vi "ex14-9.vi"() -> ()   [LabVIEW 2014]
uses:
  <vilib>/NXT/Subs/MotorOutput.ctl
  <vilib>/NXT/Dual Mode Library/Motors/MotorDistance_Single.vi
panel:
  out "X-Y二進位顯示":dbl[](array[numeric])
  out "X+Y二進位顯示":dbl[](array[numeric])
  out "X-Y":dbl
  out "X+Y":dbl
  in  "減":bool
  in  "Y":dbl
  in  "X":dbl
  out "溢位?4096":bool
  out "溢位?4096":bool
  in  "加":bool
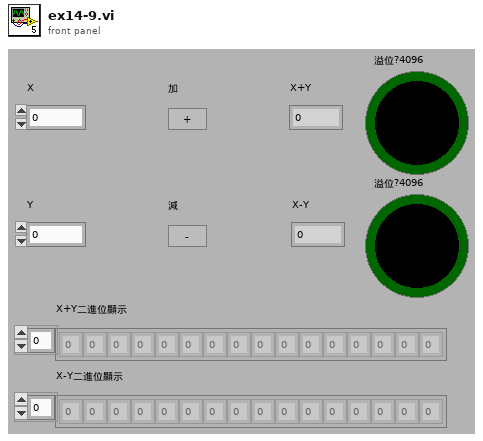
[diagram p1: front panel]
types:
  T1 = typedef "MotorOutput.ctl" = u8
  T2 = typedef "LVHSConnector.ctl" = refnum<class "BrickReference.lvclass">
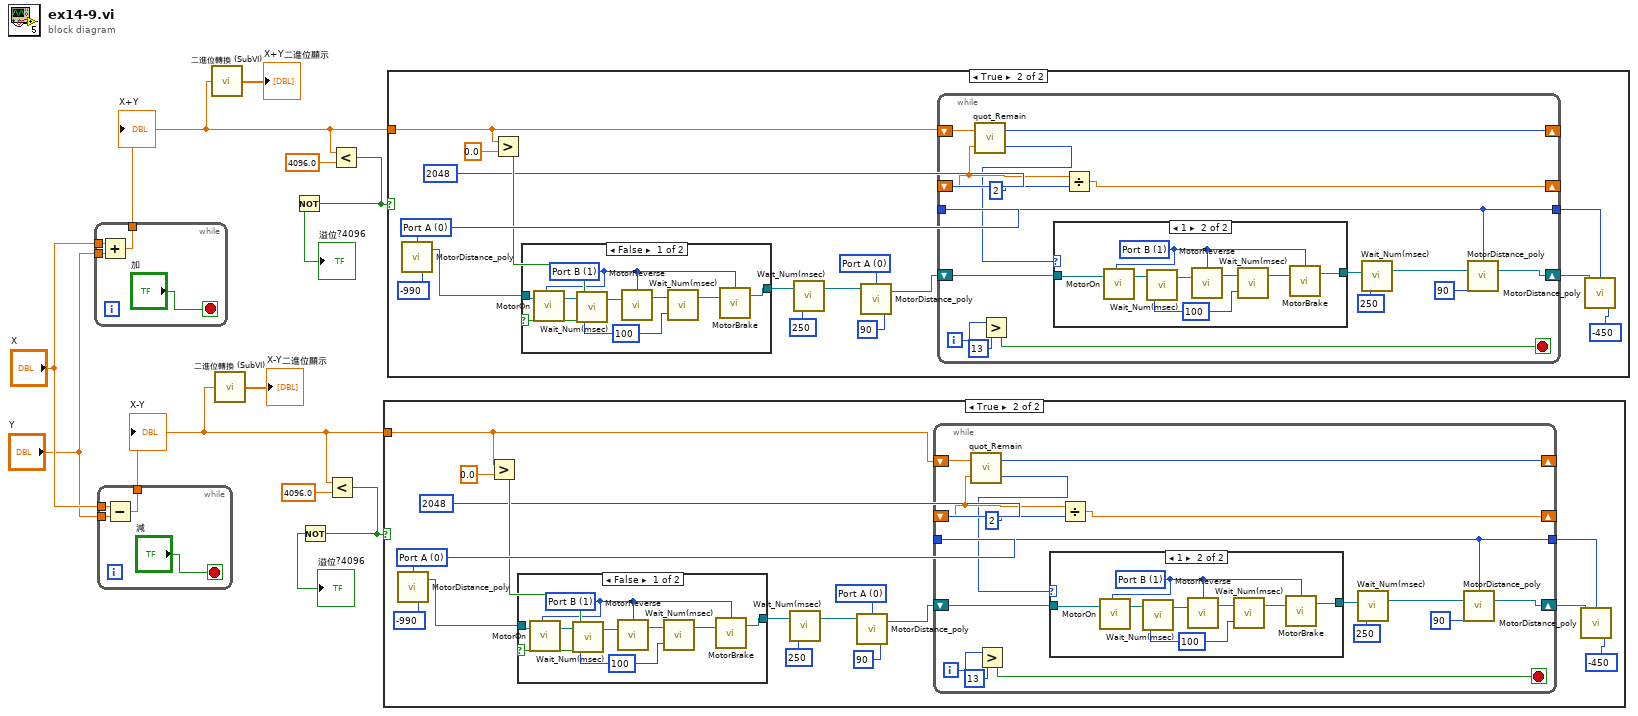
[diagram p0: block diagram]
diagram:
  n1 = while {
    tunnel: [w15] -> w4
    tunnel: "X" -> [w14]
    tunnel: "Y" -> [w13]
    stop <- "加" stop-if-true
    n2 = Add(x=w14, y=w13) -> (x+y=w15:dbl)
  }
  "X+Y" <- w4
  n3 = while {
    tunnel: [w19] -> w1
    tunnel: "X" -> [w18]
    tunnel: "Y" -> [w17]
    stop <- "減" stop-if-true
    n4 = Subtract(x=w18, y=w17) -> (x-y=w19:dbl)
  }
  "X-Y" <- w1
  n5 = call "二進位轉換 (SubVI).vi"("十進位"=w4) -> ("二進位"=→"X+Y二進位顯示":dbl[])
  n6 = call "二進位轉換 (SubVI).vi"("十進位"=w1) -> ("二進位"=→"X-Y二進位顯示":dbl[])
  n7 = Less?(x=w1, y=4096.0) -> (x < y?=w9:bool)
  n8 = Not(x=w9) -> (.not. x?=→"溢位?4096":bool)
  n9 = Less?(x=w4, y=4096.0) -> (x < y?=w11:bool)
  n10 = Not(x=w11) -> (.not. x?=→"溢位?4096":bool)
  n11 = case shown="True" w9 {
    tunnel: w1 -> [_ w21]
    frame False {
    }
    frame True {
      w23 = T1 0 items=["Port A", "Port B", "Port C", "All Ports"] ("Output Port (All Ports)")
      w33 = T1 0 items=["Port A", "Port B", "Port C", "All Ports"] ("Output Port (All Ports)")
      n12 = call-poly <vilib>:"MotorDistance_poly.vi"("Angle of Rotation (360)"=-990 ("Distance (100)"), "Output Port (All Ports)"=w33) -> ("NXT/EV3"=w29:T2)  [unwired: 2 in]
      n13 = Greater?(x=w21, y=0.0) -> (0:w30:bool)
      n14 = case shown="False" w30 {
        tunnel: w29 -> [w37 w45]
        tunnel: [w38 w45] -> w24
        frame False {
          w44 = u32 100 ("Time (100 msec)")
          w39 = T1 1 items=["Port A", "Port B", "Port C", "All Ports"] ("Output Port (All Ports)")
          n15 = call <vilib>:"MotorOn.vi"("NXT/EV3"=w37, "Output Port (All Ports)"=w39) -> ("NXT/EV3"=w43:T2)  [unwired: 2 in]
          n16 = call <vilib>:"Wait_Num(msec).vi"("Time (100 msec)"=w44, "NXT/EV3"=w43) -> ("NXT/EV3"=w42:T2)  [unwired: 2 in]
          n17 = call <vilib>:"MotorReverse.vi"("NXT/EV3"=w42, "Output Port (All Ports)"=w39) -> ("NXT/EV3"=w41:T2)  [unwired: 2 in]
          n18 = call <vilib>:"Wait_Num(msec).vi"("Time (100 msec)"=w44, "NXT/EV3"=w41) -> ("NXT/EV3"=w40:T2)  [unwired: 2 in]
          n19 = call <vilib>:"MotorBrake.vi"("NXT/EV3"=w40, "Port (All Ports)"=w39) -> ("NXT/EV3"=w38:T2)  [unwired: 2 in]
        }
        frame True {
        }
      }
      n20 = call <vilib>:"Wait_Num(msec).vi"("Time (100 msec)"=u32 250, "NXT/EV3"=w24) -> ("NXT/EV3"=w26:T2)  [unwired: 2 in]
      n21 = call-poly <vilib>:"MotorDistance_poly.vi"("Angle of Rotation (360)"=90 ("Distance (100)"), "NXT/EV3"=w26, "Output Port (All Ports)"=w23) -> ("NXT/EV3"=w22:T2)  [unwired: 1 in]
      n22 = while {
        shift-right: [w47] -> _
        shift-left: w21 -> [w49]
        shift-right: [w60] -> _
        shift-left: 2048 -> [w48]
        shift-right: [w53] -> w35
        shift-left: w22 -> [w59]
        tunnel: w33 -> [w54]
        tunnel: [w54] -> w32
        i -> [w58]
        stop <- w56 stop-if-true
        n23 = call <vilib>:"quot_Remain.vi"("y"=w48, "x"=w49) -> ("floor(x/y)"=w46:i32, "x-y*floor(x/y)"=w47:i32)
        n24 = Greater?(x=w58, y=13) -> (0:w56:bool)
        n25 = case shown="1" w46 {
          tunnel: w59 -> [w62 w64]
          tunnel: [w62 w63] -> w52
          frame 0, Default {
          }
          frame 1 {
            w65 = u32 100 ("Time (100 msec)")
            w70 = T1 1 items=["Port A", "Port B", "Port C", "All Ports"] ("Output Port (All Ports)")
            n26 = call <vilib>:"MotorOn.vi"("NXT/EV3"=w64, "Output Port (All Ports)"=w70) -> ("NXT/EV3"=w66:T2)  [unwired: 2 in]
            n27 = call <vilib>:"Wait_Num(msec).vi"("Time (100 msec)"=w65, "NXT/EV3"=w66) -> ("NXT/EV3"=w67:T2)  [unwired: 2 in]
            n28 = call <vilib>:"MotorReverse.vi"("NXT/EV3"=w67, "Output Port (All Ports)"=w70) -> ("NXT/EV3"=w68:T2)  [unwired: 2 in]
            n29 = call <vilib>:"Wait_Num(msec).vi"("Time (100 msec)"=w65, "NXT/EV3"=w68) -> ("NXT/EV3"=w69:T2)  [unwired: 2 in]
            n30 = call <vilib>:"MotorBrake.vi"("NXT/EV3"=w69, "Port (All Ports)"=w70) -> ("NXT/EV3"=w63:T2)  [unwired: 2 in]
          }
        }
        n31 = Divide(x=w48, y=2) -> (x/y=w60:dbl)
        n32 = call <vilib>:"Wait_Num(msec).vi"("Time (100 msec)"=u32 250, "NXT/EV3"=w52) -> ("NXT/EV3"=w51:T2)  [unwired: 2 in]
        n33 = call-poly <vilib>:"MotorDistance_poly.vi"("Angle of Rotation (360)"=90 ("Distance (100)"), "NXT/EV3"=w51, "Output Port (All Ports)"=w54) -> ("NXT/EV3"=w53:T2)  [unwired: 1 in]
      }
      n34 = call-poly <vilib>:"MotorDistance_poly.vi"("Angle of Rotation (360)"=-450 ("Distance (100)"), "NXT/EV3"=w35, "Output Port (All Ports)"=w32) -> ()  [unwired: 1 in, 1 out]
    }
  }
  n35 = case shown="True" w11 {
    tunnel: w4 -> [_ w71]
    frame False {
    }
    frame True {
      w73 = T1 0 items=["Port A", "Port B", "Port C", "All Ports"] ("Output Port (All Ports)")
      w83 = T1 0 items=["Port A", "Port B", "Port C", "All Ports"] ("Output Port (All Ports)")
      n36 = call-poly <vilib>:"MotorDistance_poly.vi"("Angle of Rotation (360)"=-990 ("Distance (100)"), "Output Port (All Ports)"=w83) -> ("NXT/EV3"=w79:T2)  [unwired: 2 in]
      n37 = Greater?(x=w71, y=0.0) -> (0:w80:bool)
      n38 = case shown="False" w80 {
        tunnel: w79 -> [w87 w95]
        tunnel: [w88 w95] -> w74
        frame False {
          w94 = u32 100 ("Time (100 msec)")
          w89 = T1 1 items=["Port A", "Port B", "Port C", "All Ports"] ("Output Port (All Ports)")
          n39 = call <vilib>:"MotorOn.vi"("NXT/EV3"=w87, "Output Port (All Ports)"=w89) -> ("NXT/EV3"=w93:T2)  [unwired: 2 in]
          n40 = call <vilib>:"Wait_Num(msec).vi"("Time (100 msec)"=w94, "NXT/EV3"=w93) -> ("NXT/EV3"=w92:T2)  [unwired: 2 in]
          n41 = call <vilib>:"MotorReverse.vi"("NXT/EV3"=w92, "Output Port (All Ports)"=w89) -> ("NXT/EV3"=w91:T2)  [unwired: 2 in]
          n42 = call <vilib>:"Wait_Num(msec).vi"("Time (100 msec)"=w94, "NXT/EV3"=w91) -> ("NXT/EV3"=w90:T2)  [unwired: 2 in]
          n43 = call <vilib>:"MotorBrake.vi"("NXT/EV3"=w90, "Port (All Ports)"=w89) -> ("NXT/EV3"=w88:T2)  [unwired: 2 in]
        }
        frame True {
        }
      }
      n44 = call <vilib>:"Wait_Num(msec).vi"("Time (100 msec)"=u32 250, "NXT/EV3"=w74) -> ("NXT/EV3"=w76:T2)  [unwired: 2 in]
      n45 = call-poly <vilib>:"MotorDistance_poly.vi"("Angle of Rotation (360)"=90 ("Distance (100)"), "NXT/EV3"=w76, "Output Port (All Ports)"=w73) -> ("NXT/EV3"=w72:T2)  [unwired: 1 in]
      n46 = while {
        shift-right: [w97] -> _
        shift-left: w71 -> [w99]
        shift-right: [w110] -> _
        shift-left: 2048 -> [w98]
        shift-right: [w103] -> w85
        shift-left: w72 -> [w109]
        tunnel: w83 -> [w104]
        tunnel: [w104] -> w82
        i -> [w108]
        stop <- w106 stop-if-true
        n47 = call <vilib>:"quot_Remain.vi"("y"=w98, "x"=w99) -> ("floor(x/y)"=w96:i32, "x-y*floor(x/y)"=w97:i32)
        n48 = Greater?(x=w108, y=13) -> (0:w106:bool)
        n49 = case shown="1" w96 {
          tunnel: w109 -> [w112 w114]
          tunnel: [w112 w113] -> w102
          frame 0, Default {
          }
          frame 1 {
            w115 = u32 100 ("Time (100 msec)")
            w120 = T1 1 items=["Port A", "Port B", "Port C", "All Ports"] ("Output Port (All Ports)")
            n50 = call <vilib>:"MotorOn.vi"("NXT/EV3"=w114, "Output Port (All Ports)"=w120) -> ("NXT/EV3"=w116:T2)  [unwired: 2 in]
            n51 = call <vilib>:"Wait_Num(msec).vi"("Time (100 msec)"=w115, "NXT/EV3"=w116) -> ("NXT/EV3"=w117:T2)  [unwired: 2 in]
            n52 = call <vilib>:"MotorReverse.vi"("NXT/EV3"=w117, "Output Port (All Ports)"=w120) -> ("NXT/EV3"=w118:T2)  [unwired: 2 in]
            n53 = call <vilib>:"Wait_Num(msec).vi"("Time (100 msec)"=w115, "NXT/EV3"=w118) -> ("NXT/EV3"=w119:T2)  [unwired: 2 in]
            n54 = call <vilib>:"MotorBrake.vi"("NXT/EV3"=w119, "Port (All Ports)"=w120) -> ("NXT/EV3"=w113:T2)  [unwired: 2 in]
          }
        }
        n55 = Divide(x=w98, y=2) -> (x/y=w110:dbl)
        n56 = call <vilib>:"Wait_Num(msec).vi"("Time (100 msec)"=u32 250, "NXT/EV3"=w102) -> ("NXT/EV3"=w101:T2)  [unwired: 2 in]
        n57 = call-poly <vilib>:"MotorDistance_poly.vi"("Angle of Rotation (360)"=90 ("Distance (100)"), "NXT/EV3"=w101, "Output Port (All Ports)"=w104) -> ("NXT/EV3"=w103:T2)  [unwired: 1 in]
      }
      n58 = call-poly <vilib>:"MotorDistance_poly.vi"("Angle of Rotation (360)"=-450 ("Distance (100)"), "NXT/EV3"=w85, "Output Port (All Ports)"=w82) -> ()  [unwired: 1 in, 1 out]
    }
  }
